vi "FTW-ScheduledJobset-ScheduleReadyJobs.vi"(0 "FTW Scheduled Jobset":refnum<class "FTW-ScheduledJob.lvclass">[](array[class]), 11 "error in":errorcluster) -> (4 "FTW Scheduled Jobset out":refnum<class "FTW-ScheduledJob.lvclass">[](array[class]), 6 "Scheduled Job Index to Run Now":i32=-1, 8 "Time til Next Scheduled Job":i32=-1 format="%d msec", 15 "error out":errorcluster)   [LabVIEW 2015, in "FTW-ScheduledJob.lvclass"]
uses:
  FTW-ScheduledJob.lvclass
panel:
  # "Inputs"
  # "Outputs"
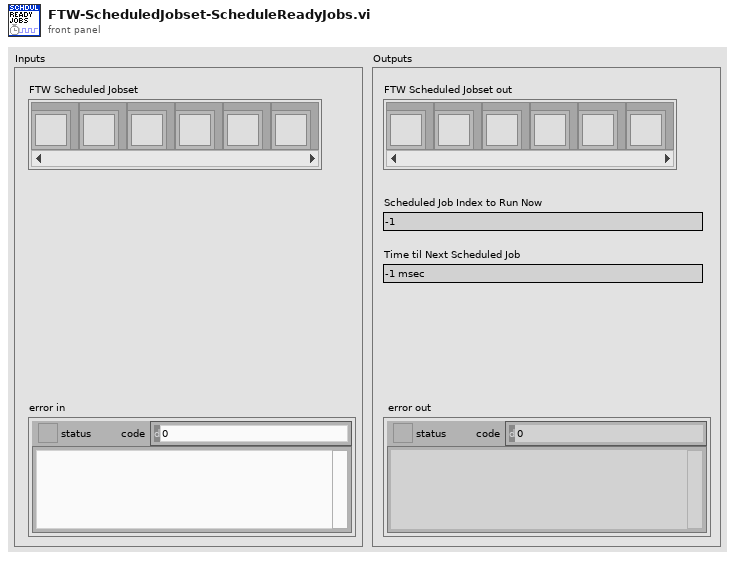
[diagram p1: front panel]
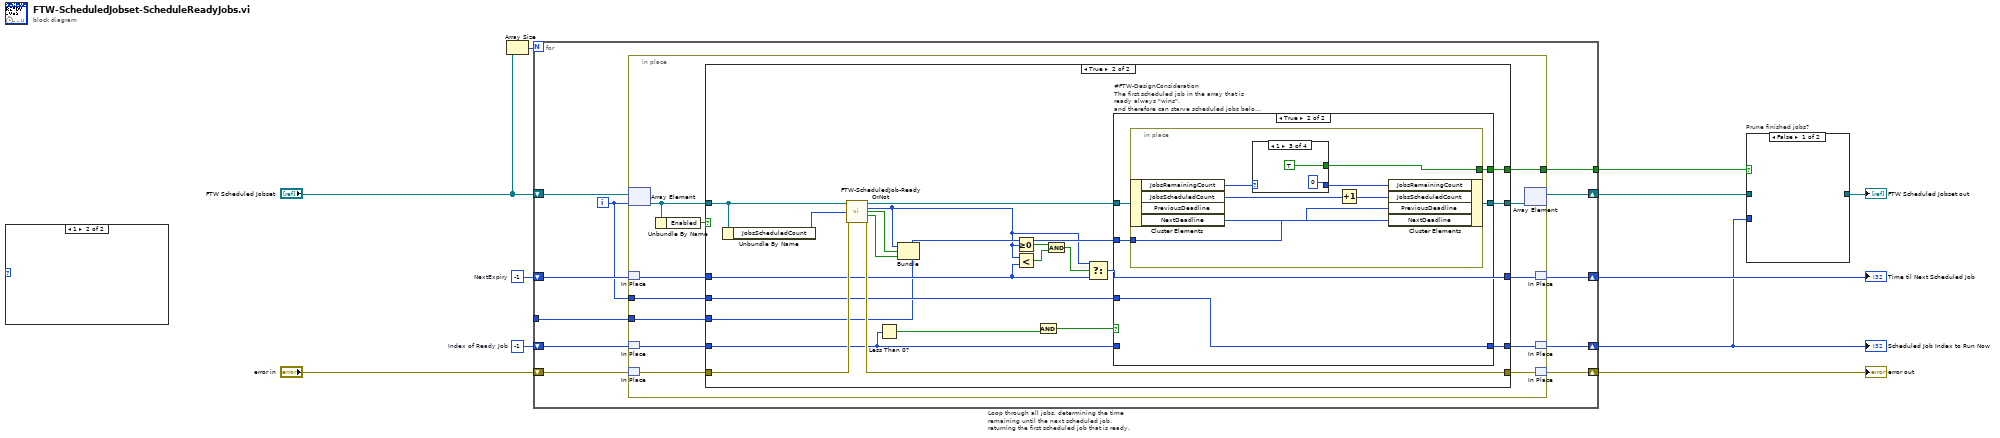
[diagram p0: block diagram]
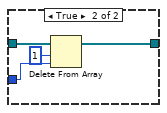
[diagram p2: hidden frame]
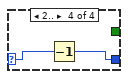
[diagram p8: hidden frame]
diagram:
  w5 = -1  # Index of Ready Job
  w7 = -1  # NextExpiry
  n1 = case shown="1" {
    selector: _ -> [_ _]
    frame -1 {
    }
    frame 1 {
    }
  }
  n2 = Array Size(array="FTW Scheduled Jobset") -> (size(s)=w9:i32)
  n3 = for "Loop through all jobs, determining the time remaining until the next scheduled job, returning the first scheduled job that is ready." {
    N: w9 -> [_]
    shift-right: [w20] -> w3
    shift-left: "FTW Scheduled Jobset" -> [w21]
    shift-right: [w19] -> w8
    shift-left: "error in" -> [w22]
    shift-right: [w17] -> w6
    shift-left: w7 -> [w18]
    shift-right: [w15] -> w2
    shift-left: w5 -> [w16]
    tunnel: _ -> [w13]
    tunnel: [w12] -> w4
    i -> [w14]
    n4 = in-place {
      in-place-border: w14 -> [w25]
      in-place-border: w13 -> [w24]
      in-place-border: [w23] -> w12
      n5 = in-place-array #1(w21, w14) -> (w29:refnum<class "FTW-ScheduledJob.lvclass">)
      n6 = in-place-match #2(w18) -> (w31:i32)
      n7 = in-place-match #3(w16) -> (w27:i32)
      n8 = in-place-match #4(w22) -> (w34:errorcluster)
      n9 = Unbundle By Name(w29) -> ("Enabled"=w28:bool)
      n10 = case shown="True" w28 {
        tunnel: w34 -> [w36 w59]
        tunnel: [w38 w53] -> w33
        tunnel: [w36 w58] -> w32
        tunnel: w31 -> [w37 w55]
        tunnel: [w37 w54] -> w30
        tunnel: w29 -> [w38 w47]
        tunnel: w27 -> [w35 w50]
        tunnel: [w35 w49] -> w26
        tunnel: w25 -> [_ w48]
        tunnel: w24 -> [_ w44]
        tunnel: [_ w45] -> w23
        frame False {
        }
        frame True {
          n11 = Unbundle By Name(w47) -> ("JobsScheduledCount"=w42:i32)
          n12 = call-dynamic "FTW-ScheduledJob-ReadyOrNot.vi"("FTW Scheduled Job"=w47, 7:w42, "error in"=w59) -> ("FTW Scheduled Job out"=w43:refnum<class "FTW-ScheduledJob.lvclass">, "Next Schedule Deadline"=w41:u32, "Next Schedule Active"=w40:bool, "Ready to Schedule"=w39:bool, "error out"=w58:errorcluster)  [unwired: 8 in]
          n13 = Less Than 0?(x=w50) -> (x < 0?=w52:bool)
          n14 = Bundle("Next Schedule Deadline"=w41, "Next Schedule Active"=w40, "Ready to Schedule"=w39) -> ()  [unwired: 1 in, 1 out]
          n15 = Greater Or Equal To 0?(x=w41) -> (x >= 0?=w46:bool)
          n16 = Less?(x=w41, y=w55) -> (x < y?=w57:bool)
          n17 = And(y=w52) -> (x .and. y?=w51:bool)  [unwired: 1 in]
          n18 = And(x=w46, y=w57) -> (x .and. y?=w56:bool)
          n19 = Select(t=w41, s=w56, f=w55) -> (s? t:f=w54:u32)
          n20 = case "#FTW-DesignConsideration\nThe first scheduled job in the array that is ready always \"wins\",\nand therefore can starve scheduled jobs below it in the array." shown="True" w51 {
            tunnel: [w60 w64] -> w53
            tunnel: w43 -> [w60 w65]
            tunnel: w50 -> [w61 _]
            tunnel: [w61 w66] -> w49
            tunnel: w48 -> [_ w66]
            tunnel: w44 -> [_ w63]
            tunnel: [_ w62] -> w45
            frame False {
            }
            frame True {
              n21 = in-place {
                in-place-border: w63 -> [w73]
                in-place-border: [w69] -> w62
                n22 = in-place-cluster #5(w65) -> ("JobsRemainingCount"=w71:i32, "JobsScheduledCount"=w68:i32, "NextDeadline"=w72:u32)  [unwired: 1 out]
                n23 = case shown="1" w71 {
                  selector: w71 -> [w74 w75 _ w79]
                  tunnel: [w74 w75 0 ("ScheduleCountRemaining") w78] -> w70
                  tunnel: [_ _ TRUE _] -> w69
                  frame -1 {
                    # "Loop forever."
                  }
                  frame Default {
                    # "This should\nnever happen."
                  }
                  frame 1 {
                  }
                  frame 2.. {
                    n24 = Decrement(x=w79) -> (x-1=w78:i32)
                  }
                }
                n25 = Increment(x=w68) -> (x+1=w67:i32)
                n26 = in-place-cluster #5("JobsRemainingCount"=w70, "JobsScheduledCount"=w67, "PreviousDeadline"=w72, "NextDeadline"=w73) -> (w64:refnum<class "FTW-ScheduledJob.lvclass">)
              }
            }
          }
        }
      }
      n27 = in-place-array #1(w33) -> (w20:refnum<class "FTW-ScheduledJob.lvclass">[])  [unwired: 1 out]
      n28 = in-place-match #2(w30) -> (w17:i32)
      n29 = in-place-match #3(w26) -> (w15:i32)
      n30 = in-place-match #4(w32) -> (w19:errorcluster)
    }
  }
  "error out" <- w8
  "Time til Next Scheduled Job" <- w6
  "Scheduled Job Index to Run Now" <- w2
  n31 = case "Prune finished jobs?" shown="False" w4 {
    tunnel: w3 -> [_ w83]
    tunnel: w2 -> [_ w80]
    tunnel: [_ w82] -> w1
    frame False {
    }
    frame True {
      n32 = Delete From Array(array=w83, length=1, index=w80) -> (array with subset deleted=w82:refnum<class "FTW-ScheduledJob.lvclass">[])  [unwired: 1 out]
    }
  }
  "FTW Scheduled Jobset out" <- w1
